vi "Exit.vi"(7 "Exit Notifier":refnum<notifier>, 8 "error in (no error)":errorcluster, 11 "UI Queue":refnum<queue>) -> (0 "error out":errorcluster)   [LabVIEW 2015, in "PL Model.lvlib"]
uses:
  PL Model.lvlib
  support/Message Queue/Message Queue.lvlib
  support/Message Queue/Message Cluster.ctl
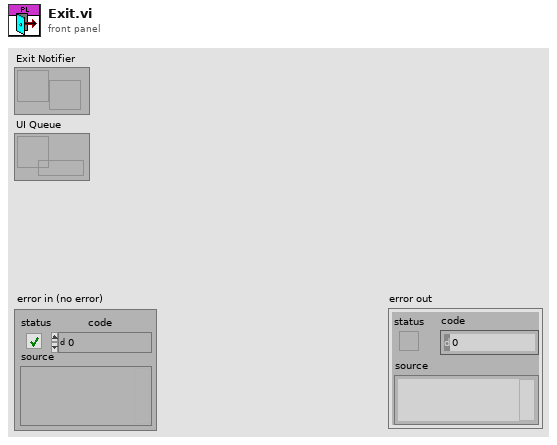
[diagram p1: front panel]
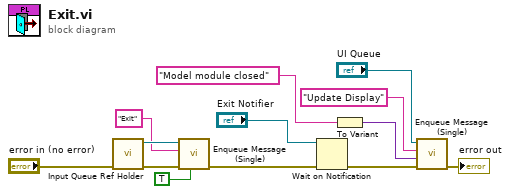
[diagram p0: block diagram]
diagram:
  n1 = call "Input Queue Ref Holder.vi"("error in (no error)"="error in (no error)") -> ("error out"=w13:errorcluster, "Input Message Queue"=w11:refnum<queue>)  [unwired: 9 in]
  n2 = call "Enqueue Message (Single).vi"("Priority Message? (F)"=TRUE, "error in (no error)"=w13, "Message"="Exit", "Message Queue"=w11) -> ("error out"=w9:errorcluster)  [unwired: 6 in, 1 out]
  n3 = Wait on Notification(notifier="Exit Notifier", error in (no error)=w9) -> (error out=w7:errorcluster)  [unwired: 2 in, 3 out]
  n4 = To Variant(anything="Model module closed" ("Message")) -> (Variant=w2:variant)
  n5 = call "Enqueue Message (Single).vi"("error in (no error)"=w7, "Message Data"=w2, "Message"="Update Display", "Message Queue"="UI Queue") -> ("error out"=→"error out":errorcluster)  [unwired: 6 in, 1 out]
